vi "ReadGasData Example.vi"() -> ()   [LabVIEW 2019]
uses:
  BrooksDLL.dll
panel:
  out "Flow Unit Comment":string
  out "Flow Range":sgl format="%.2f"
  out "Flow Unit Code":u8
  out "Ref Pressure Unit Comment":string
  out "Ref Pressure":sgl format="%.2f"
  out "Ref Pressure Unit":u8
  out "Ref Temp Unit Comment":string
  out "Ref Temp":sgl format="%.2f"
  out "Ref Temp Unit":u8
  out "Density Code Comment":string
  out "Density":sgl format="%.2f"
  out "Density Code":u8
  in  "GasNumber":u8(ring) items=["1", "2", "3", "4", "5", "6", "7", "8", "9", "10"]
  out "S2 String":string
  out "S1 String":string
  out "S2":u8 format="%.0x"
  out "S1":u8 format="%.0x"
  out "Function Output Comment":string
  out "output param":i32
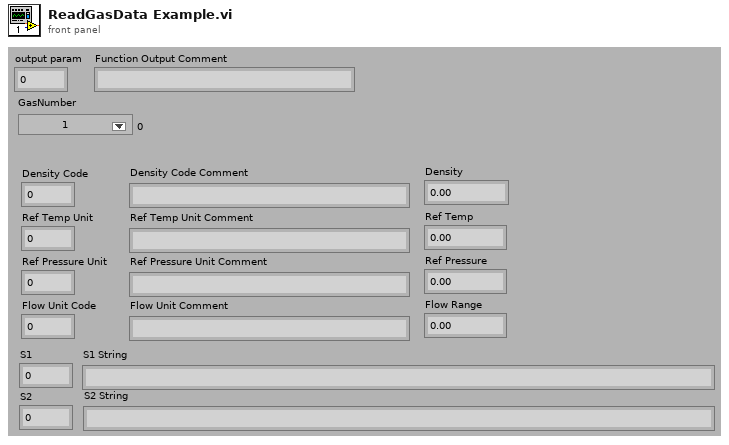
[diagram p1: front panel]
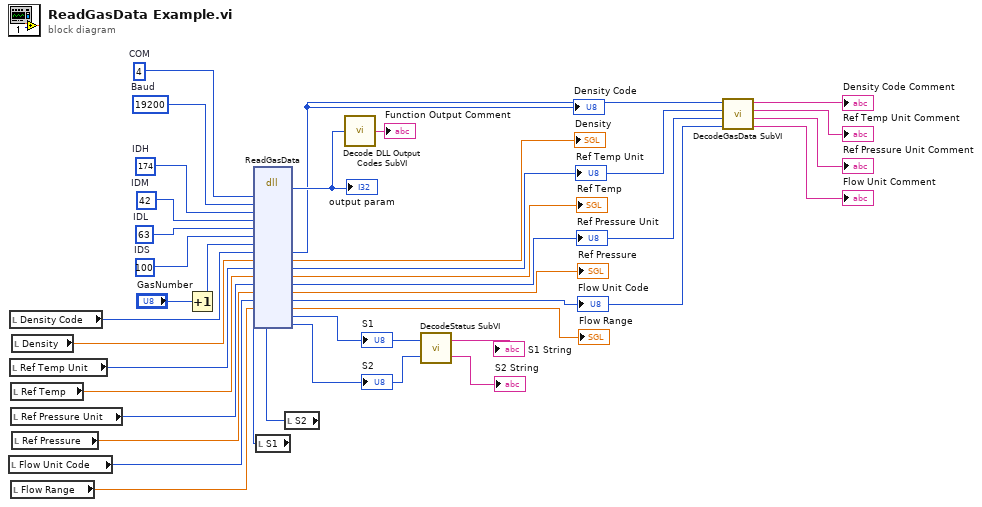
[diagram p0: block diagram]
diagram:
  w31 = u8 100  # IDS
  w32 = u8 63  # IDL
  w33 = u8 42  # IDM
  w34 = u8 174  # IDH
  w35 = 19200  # Baud
  w36 = 4  # COM
  n1 = local read "Flow Unit Code"() -> (w14:u8)
  n2 = local read "Density Code"() -> (w20:u8)
  n3 = local read "Ref Temp Unit"() -> (w18:u8)
  n4 = local read "Ref Temp"() -> (w17:sgl)
  n5 = local read "Ref Pressure Unit"() -> (w16:u8)
  n6 = local read "Flow Range"() -> (w13:sgl)
  n7 = local read "Density"() -> (w19:sgl)
  n8 = local read "Ref Pressure"() -> (w15:sgl)
  n9 = Increment(x="GasNumber") -> (x+1=w21:u8)
  n10 = local read "S1"() -> (w23:u8)
  n11 = local read "S2"() -> (w24:u8)
  n12 = dll-call lib="G:/Developpement_de_Programmes/Programmes/Controle de pression/164J027_AD/Brooks DLL 1.0.1.0 32bit/Brooks DLL 1.0.1.0 Release 10032016/S Protocol/BrooksDLL.dll" fn="ReadGasData"("COM"=w36, "Baud"=w35, "IDH"=w34, "IDM"=w33, "IDL"=w32, "IDS"=w31, "GasNumber"=w21, "DensityCode"=w20, "Density"=w19, "RefTempUnit"=w18, "RefTemp"=w17, "RefPressureUnit"=w16, "RefPressure"=w15, "FlowUnitCode"=w14, "FlowRange"=w13, "S1"=w23, "S2"=w24) -> (w30:i32, "DensityCode"=w8:u8, "Density"=→"Density":sgl, "RefTempUnit"=w7:u8, "RefTemp"=→"Ref Temp":sgl, "RefPressureUnit"=w6:u8, "RefPressure"=→"Ref Pressure":sgl, "FlowUnitCode"=w5:u8, "FlowRange"=→"Flow Range":sgl, "S1"=w25:u8, "S2"=w26:u8)  [unwired: 10 in, 2 out]
  "output param" <- w30
  "S1" <- w25
  "S2" <- w26
  "Density Code" <- w8
  "Ref Temp Unit" <- w7
  "Ref Pressure Unit" <- w6
  "Flow Unit Code" <- w5
  n13 = call "Decode DLL Output Codes SubVI.vi"("Numeric"=w30) -> ("Function Output Comment"=→"Function Output Comment":string)
  n14 = call "DecodeStatus SubVI.vi"("S2"=w26, "S1"=w25) -> ("S2 String"=→"S2 String":string, "S1 String"=→"S1 String":string)
  n15 = call "DecodeGasData SubVI.vi"("FlowUnit"=w5, "Re fPressureUnit"=w6, "RefTempUnit"=w7, "DensityUnitCode"=w8) -> ("Flow Unit Comment"=→"Flow Unit Comment":string, "Ref Pressure Unit Comment"=→"Ref Pressure Unit Comment":string, "Temperature Unit Comment"=→"Ref Temp Unit Comment":string, "Density Unit Comment"=→"Density Code Comment":string)
